vi "closeWMPRef.vi"(8 "error in (no error)":errorcluster, 11 "SoundAO in":refnum<class "SoundAO.lvclass">) -> (0 "error out":errorcluster, 3 "SoundAO out":refnum<class "SoundAO.lvclass">)   [LabVIEW 2011, in "Hardware.lvlib" / "Channels.lvlib" / "SoundAO.lvclass"]
uses:
  SoundAO.lvclass
  SoundAO.lvclass/SoundAO.ctl
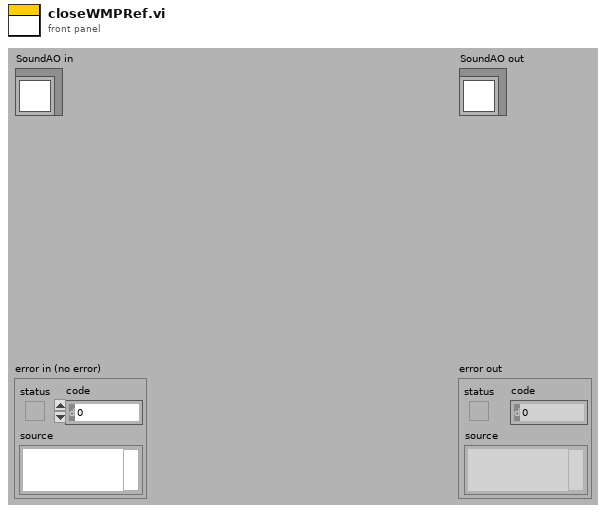
[diagram p1: front panel]
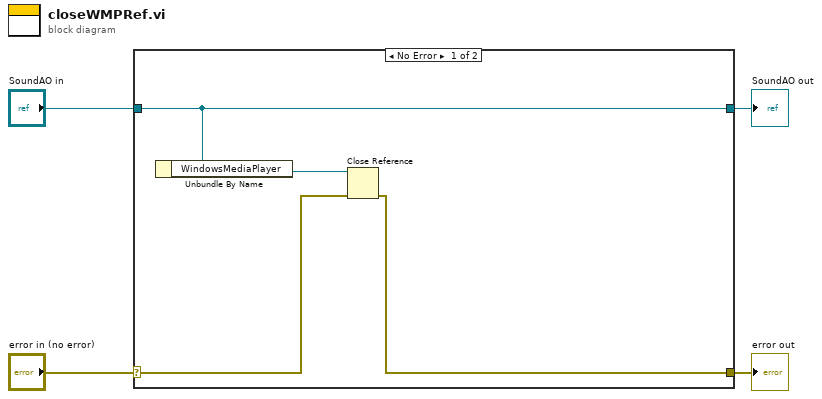
[diagram p0: block diagram]
diagram:
  n1 = case shown="No Error" "error in (no error)" {
    selector: "error in (no error)" -> [w6 w10]
    tunnel: [w5 w10] -> w3
    tunnel: [w8 w9] -> w1
    tunnel: "SoundAO in" -> [w8 w9]
    frame No Error {
      n2 = Unbundle By Name(w8) -> ("WindowsMediaPlayer"=w7:refnum<k7>)
      n3 = Close Reference(reference=w7, error in (no error)=w6) -> (error out=w5:errorcluster)
    }
    frame Error {
    }
  }
  "error out" <- w3
  "SoundAO out" <- w1
